vi "read reverse power dBm.vi"(0 "VISA resource name":refnum<visa-resource-name>="GPIB0::12::INSTR", 1 "error in (no error)":errorcluster) -> (2 "VISA resource name out":refnum<visa-resource-name>, 3 "reverse power (dBm)":dbl, 4 "error out":errorcluster)   [LabVIEW 2009, in "MicrowaveAmplifier.lvlib"]
uses:
  MicrowaveAmplifier.lvlib
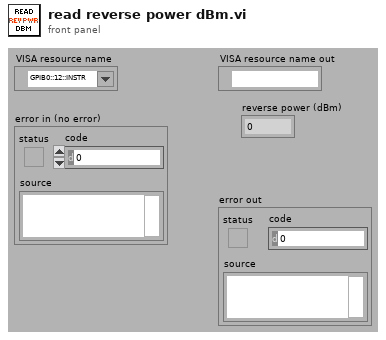
[diagram p1: front panel]
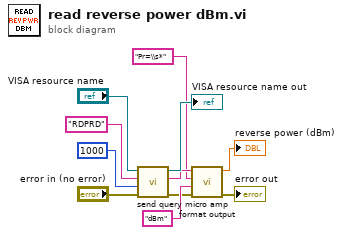
[diagram p0: block diagram]
diagram:
  n1 = call "send query micro amp.vi"("error in (no error)"="error in (no error)", "Bytes Count"=u32 1000 ("bytes to read (1000) 2"), "write buffer"="RDPRD" ("write buffer 2"), "VISA resource name"="VISA resource name") -> ("error out"=w4:errorcluster, "read buffer"=w2:string, "VISA resource name out"=→"VISA resource name out":refnum<visa-resource-name>)  [unwired: 5 in]
  n2 = call "format output.vi"("error in (no error)"=w4, "Search for String"="dBm" ("search string"), "Regular Expression"="Pr=\\s*" ("search string"), "Input String"=w2) -> ("error out"=→"error out":errorcluster, "Output"=→"reverse power (dBm)":dbl)  [unwired: 6 in]
